vi "T7 Actual Scan Rate KAG.vi"() -> ()   [LabVIEW 2022 SP3]
doc: "This VI does not work. Tried to calculate and actual sample rate (according to the T7 core timer). Couldn't get it to work. Gave up."
uses:
  <vilib>/Analysis/baseanly.llb/Mean (DBL).vi
  <vilib>/Analysis/NI_AALBase.lvlib
panel:
  out "Max ?":dbl
  in  "Numeric":u32
  out "(hi.lo) time?":dbl[](array[numeric])
  out "Scan Something":dbl
  out "error":i32
  out "mean":dbl format="%0.2f"
  out "x-y":dbl[](array[numeric]) format="%.3e"
  out "array (last n elements first)":u32[](array[numeric])
  out "(hi.lo)":u32[](array[numeric])
  out "subarray":u16[][](array[numeric])
  out "size(s)":i32[](array[numeric])
  in  "error in":errorcluster
  out "error out":errorcluster
  in  "Byte Data":u16[][](array[numeric])
  # "Never did turn this into anything meaningful. Not sure what I am getting out of streaming the core timer.\nWhat do the integer values mean? The CORE_TIMER is a UINT32 value so the maximum is 4,294,967,296.  It cycles through this value back to 0 (presumably). Not sure but I think that the timer increments by 1 for every 2 pulses of the core clock (~80MHz). This means that the timer values should reset according to the following quotient:\n\nU32      4,294,967,296   ticks\n---------------------------   =    107.374  seconds\ntimer         40,000,000     Hz\n\nWell, I was sampling at a high rate, and the tick counter was certainly resetting quicker than that.\nFurthermore, this really only gives the actual sample rate \"according to the T7\"\n\nUltimately, I undid the mods I made to other VIs that made this VI go. (That is to say that I removed the CORE_TIMER & STREAM_DATA_CAPTURE_16 (16-bit overflow) from the scan table. There were several places where small adjustments needed to be made to handle the addition of these two channels. Some of those comments are still in the place where the mods used to be. But having given up on this bit, I have removed the mods."
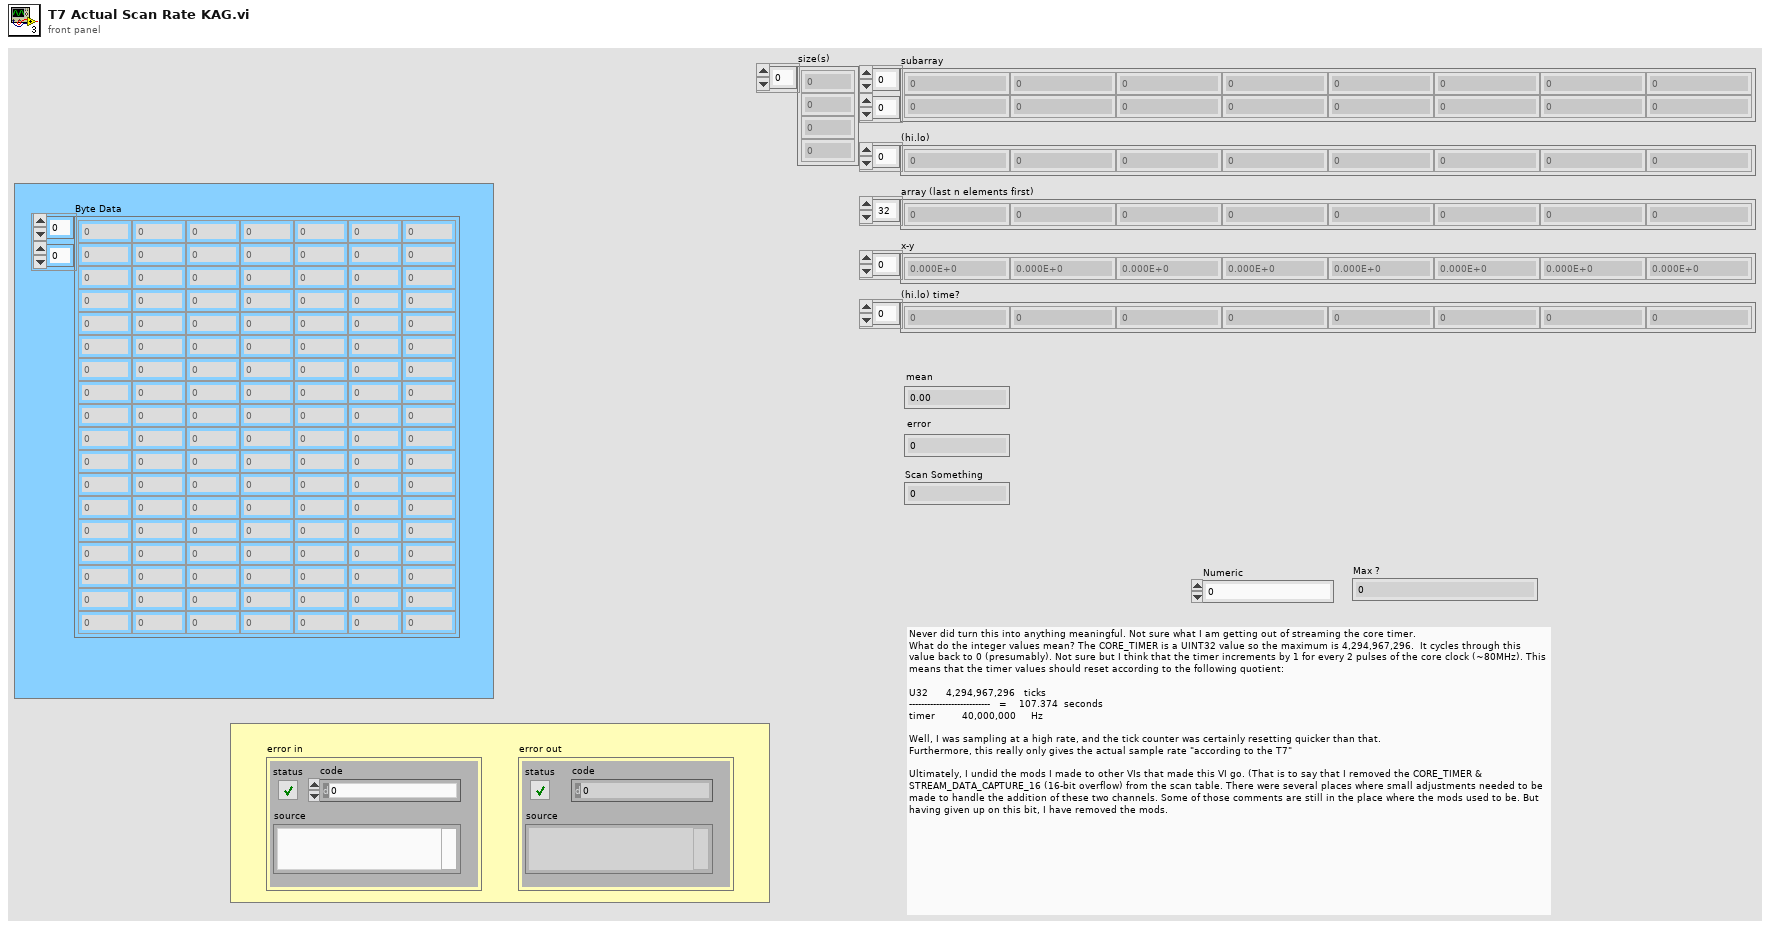
[diagram p1: front panel]
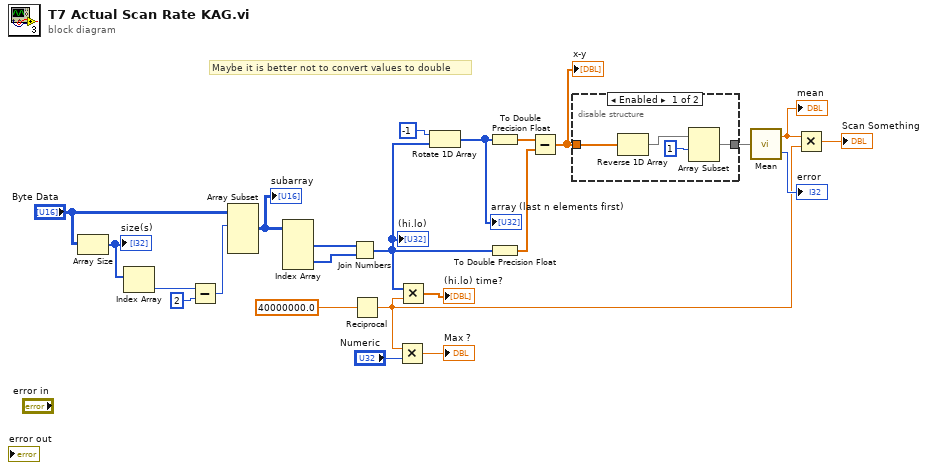
[diagram p0: block diagram]
diagram:
  # "Maybe it is better not to convert values to double"
  n1 = Array Size(array="Byte Data") -> (size(s)=w22:i32[])
  "size(s)" <- w22
  n2 = Index Array(array=w22) -> (element=w21:i32)  [unwired: 1 in]
  n3 = Subtract(x=w21, y=2) -> (x-y=w19:i32)
  n4 = Array Subset(array="Byte Data", index (row)=w19) -> (w18:u16[][])  [unwired: 3 in]
  "subarray" <- w18
  n5 = Index Array(array=w18) -> (element #1=w17:u16[], element #2=w16:u16[])  [unwired: 4 in]
  n6 = Join Numbers(hi=w17, lo=w16) -> ((hi.lo)=w7:u32[])
  "(hi.lo)" <- w7
  n7 = Reciprocal(x=40000000.0) -> (1/x=w4:dbl)
  n8 = Multiply(x=w4, y="Numeric") -> (x*y=→"Max ?":dbl)
  n9 = Multiply(x=w7, y=w4) -> (x*y=→"(hi.lo) time?":dbl[])
  n10 = Rotate 1D Array(1:w7, 2:-1 ("n")) -> (0:w14:u32[])
  "array (last n elements first)" <- w14
  n11 = To Double Precision Float(number=w14) -> (double precision float=w1:dbl[])
  n12 = To Double Precision Float(number=w7) -> (double precision float=w2:dbl[])
  n13 = Subtract(x=w1, y=w2) -> (x-y=w9:dbl[])
  "x-y" <- w9
  n14 = disable-structure shown="Enabled" {
    disable-tunnel: w9 -> [w27 w28]
    disable-tunnel: [w24 w28] -> w8
    frame Enabled {
      n15 = Reverse 1D Array(array=w27) -> (reversed array=w26:dbl[])
      n16 = Array Subset(array=w26, index=1) -> (w24:dbl[])  [unwired: 1 in]
    }
    frame Disabled {
    }
  }
  n17 = call-poly <vilib>:"Mean.vi"("X"=w8) -> ("mean"=w12:dbl, "error"=→"error":i32)
  "mean" <- w12
  n18 = Multiply(x=w12, y=w4) -> (x*y=→"Scan Something":dbl)
